vi "HEX IP ADRES.vi"(2 "IP Address":string) -> (6 "IP Address ASCII":string, 7 "IP Address HEX":string)   [LabVIEW 2017]
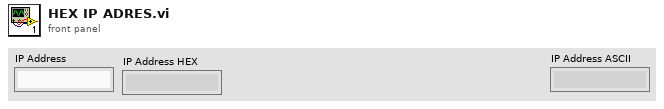
[diagram p1: front panel]
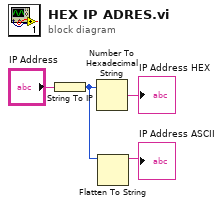
[diagram p0: block diagram]
diagram:
  n1 = String To IP(1:"IP Address") -> (0:w2:u32)
  n2 = Number To Hexadecimal String(2:w2) -> (0:→"IP Address HEX":string)  [unwired: 1 in]
  n3 = Flatten To String(anything=w2) -> (data string=→"IP Address ASCII":string)  [unwired: 3 in, 2 out]
